vi "generateEventStatusChecks.vi"(8 "error in (no error)":errorcluster, 10 "EventStatusChecks":T1, 11 "UserEvents in":refnum<class "UserEvents.lvclass">) -> (0 "error out":errorcluster, 3 "UserEvents out":refnum<class "UserEvents.lvclass">)   [LabVIEW 2016, in "UserEvents.lvclass"]
uses:
  UserEvents.lvclass
  DataTypes/Topics/EventStatusChecks.ctl
  DataTypes/Topics/Parts/Timestamp.ctl
  UserEvents.lvclass/UserEvents.ctl
  DataTypes/Topics/M1M3SupportTopics.lvlib
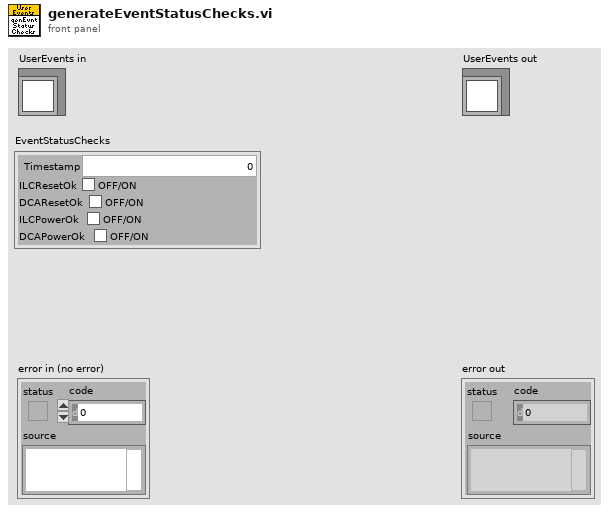
[diagram p1: front panel]
types:
  T1 = typedef "M1M3SupportTopics.lvlib/EventStatusChecks.ctl" = cluster{"Timestamp":T2, "ILCResetOk":bool, "DCAResetOk":bool, "ILCPowerOk":bool, "DCAPowerOk":bool}
  T2 = typedef "M1M3SupportTopics.lvlib/Timestamp.ctl" = dbl
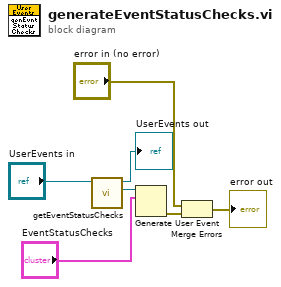
[diagram p0: block diagram]
diagram:
  n1 = call "getEventStatusChecks.vi"("UserEvents in"="UserEvents in") -> ("EventStatusChecks"=w7:refnum<user-event>, "UserEvents out"=→"UserEvents out":refnum<class "UserEvents.lvclass">)  [unwired: 9 in]
  n2 = Generate User Event(user event=w7, event data cluster="EventStatusChecks") -> (error out=w4:errorcluster)  [unwired: 2 in, 1 out]
  n3 = Merge Errors("error in (no error)", w4) -> (→"error out":errorcluster)
